vi "Enqueue Test Cases to Slave Runners.vi"(8 "error in (no error)":errorcluster, 10 "Test Cases":refnum<class "LUnit Test Case.lvclass">[](array[class]), 11 "Test Runner in":refnum<class "Test Runner.lvclass">) -> (0 "error out":errorcluster, 2 "Schedule":i32[](array[numeric]), 3 "Test Runner out":refnum<class "Test Runner.lvclass">)   [LabVIEW 2020, in "Test Runner.lvclass"]
uses:
  Test Runner.lvclass
  Slave Test Runner/Slave Test Runner.lvclass
  Test Case/LUnit Test Case.lvclass
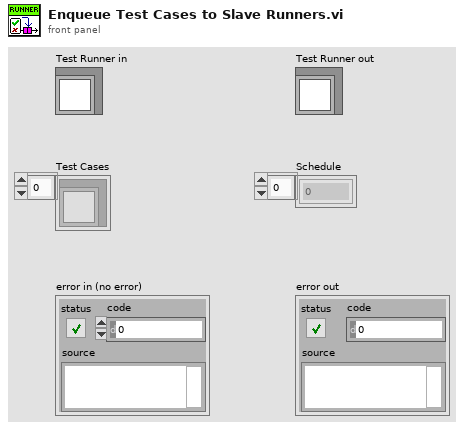
[diagram p1: front panel]
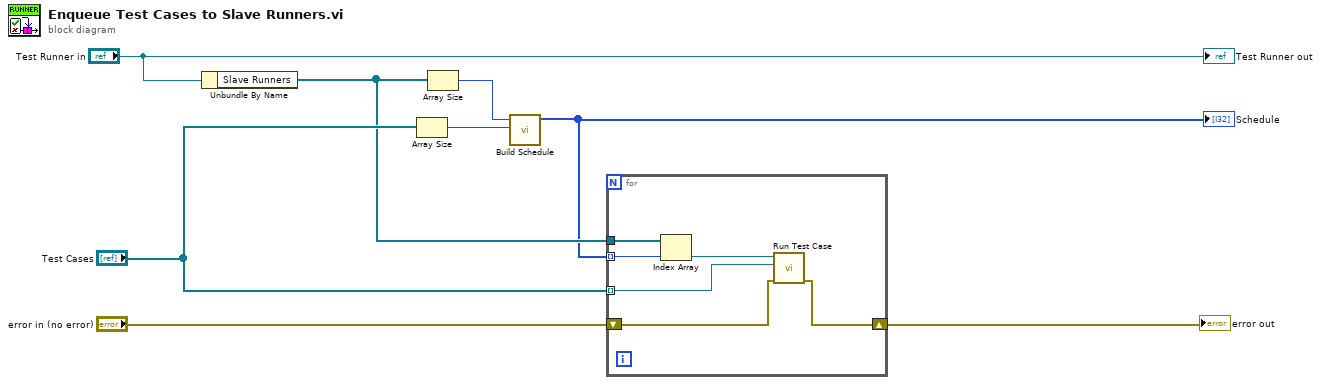
[diagram p0: block diagram]
diagram:
  n1 = Unbundle By Name("Test Runner in") -> ("Slave Runners"=w5:refnum<class "Slave Test Runner.lvclass">[])
  n2 = Array Size(array="Test Cases") -> (size(s)=w3:i32)
  n3 = Array Size(array=w5) -> (size(s)=w7:i32)
  n4 = call "Build Schedule.vi"("Number of Test Cases"=w3, "Number of Test Runners"=w7) -> ("Schedule"=w2:i32[])  [unwired: 9 in]
  "Schedule" <- w2
  n5 = for {
    tunnel: w2 -> [w13] mode=indexing
    tunnel: "Test Cases" -> [w11] mode=indexing
    tunnel: w5 -> [w14]
    shift-right: [w9] -> w1
    shift-left: "error in (no error)" -> [w10]
    n6 = Index Array(array=w14, index=w13) -> (element=w12:refnum<class "Slave Test Runner.lvclass">)
    n7 = call "Run Test Case.vi"("error in (no error)"=w10, "Test Case"=w11, "Slave Test Runner In"=w12) -> ("error out"=w9:errorcluster)  [unwired: 7 in, 1 out]
  }
  "error out" <- w1
  "Test Runner out" <- "Test Runner in"
